vi "SendXML.vi"(2 "Send":string, 3 "URI in":string) -> (0 "error out":errorcluster, 1 "Reply":string)   [LabVIEW 2010]
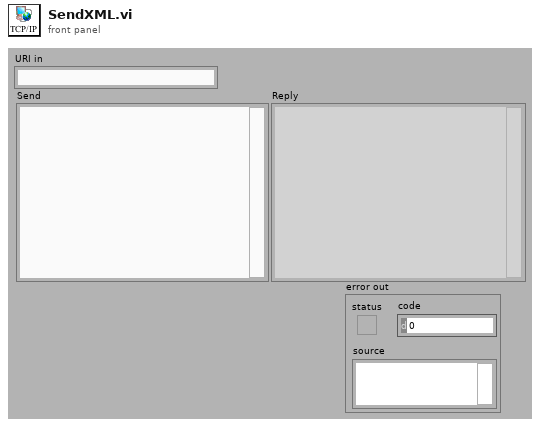
[diagram p1: front panel]
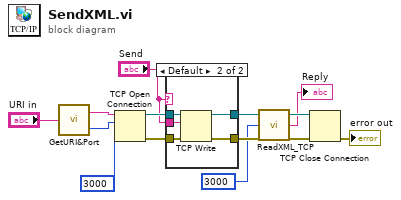
[diagram p0: block diagram]
diagram:
  n1 = call "GetURI&Port.vi"("URI in"="URI in") -> ("Port"=w14:u16, "URI"=w13:string)
  n2 = TCP Open Connection(address=w13, remote port or service name=w14, timeout ms (60000)=3000) -> (connection ID=w11:refnum<k5>, error out=w12:errorcluster)  [unwired: 2 in]
  n3 = case shown="Default" "Send" {
    tunnel: w12 -> [w15 w21]
    tunnel: w11 -> [w16 w20]
    tunnel: [w16 w19] -> w10
    tunnel: [w15 w18] -> w9
    tunnel: "Send" -> [_ w17]
    frame "" {
    }
    frame Default {
      n4 = TCP Write(connection ID=w20, data in=w17, error in (no error)=w21) -> (connection ID out=w19:refnum<k5>, error out=w18:errorcluster)  [unwired: 1 in, 1 out]
    }
  }
  n5 = call "ReadXML_TCP.vi"("error in"=w9, "timeout ms (3000)"=3000 ("timeout ms (25000)"), "connection ID in"=w10) -> ("error out"=w7:errorcluster, "data out"=→"Reply":string, "connection ID out"=w6:refnum<k5>)
  n6 = TCP Close Connection(connection ID=w6, error in (no error)=w7) -> (error out=→"error out":errorcluster)  [unwired: 1 in, 1 out]
